vi "Test - Draw Teapot.vi"() -> ()   [LabVIEW 2022 SP3, in "Raster.lvlib"] (continued)
3"={"Position"={"x"=314.33466, "y"=375.0982, "z"=0.9916978}, "UV"={"u"=0.0, "v"=0.0}, "Colour"=12517256}, "Alpha"=0.0, "Alpha Blending Enabled"=FALSE, "Colour"=10409073}, {"Vertex 1"={"Position"={"x"=470.44748, "y"=365.30457, "z"=0.99189657}, "UV"={"u"=0.0, "v"=0.0}, "Colour"=12517256}, "Vertex 2"={"Position"={"x"=469.86905, "y"=368.43405, "z"=0.9918814}, "UV"={"u"=0.0, "v"=0.0}, "Colour"=12517256}, "Vertex 3"={"Position"={"x"=485.44525, "y"=370.00763, "z"=0.99169356}, "UV"={"u"=0.0, "v"=0.0}, "Colour"=12517256}, "Alpha"=0.0, "Alpha Blending Enabled"=FALSE, "Colour"=2964768}, {"Vertex 1"={"Position"={"x"=469.71655, "y"=372.48022, "z"=0.9918774}, "UV"={"u"=0.0, "v"=0.0}, "Colour"=12517256}, "Vertex 2"={"Position"={"x"=470.04498, "y"=373.40598, "z"=0.991886}, "UV"={"u"=0.0, "v"=0.0}, "Colour"=12517256}, "Vertex 3"={"Position"={"x"=485.66537, "y"=375.0982, "z"=0.9916978}, "UV"={"u"=0.0, "v"=0.0}, "Colour"=12517256}, "Alpha"=0.0, "Alpha Blending Enabled"=FALSE, "Colour"=10540914}, {"Vertex 1"={"Position"={"x"=329.95502, "y"=373.40598, "z"=0.991886}, "UV"={"u"=0.0, "v"=0.0}, "Colour"=12517256}, "Vertex 2"={"Position"={"x"=330.28342, "y"=372.48022, "z"=0.9918774}, "UV"={"u"=0.0, "v"=0.0}, "Colour"=12517256}, "Vertex 3"={"Position"={"x"=314.74542, "y"=374.1431, "z"=0.9916899}, "UV"={"u"=0.0, "v"=0.0}, "Colour"=12517256}, "Alpha"=0.0, "Alpha Blending Enabled"=FALSE, "Colour"=10540914}, {"Vertex 1"={"Position"={"x"=330.35867, "y"=370.8254, "z"=0.9918754}, "UV"={"u"=0.0, "v"=0.0}, "Colour"=12517256}, "Vertex 2"={"Position"={"x"=330.13095, "y"=368.43405, "z"=0.9918814}, "UV"={"u"=0.0, "v"=0.0}, "Colour"=12517256}, "Vertex 3"={"Position"={"x"=314.55475, "y"=370.00763, "z"=0.99169356}, "UV"={"u"=0.0, "v"=0.0}, "Colour"=12517256}, "Alpha"=0.0, "Alpha Blending Enabled"=FALSE, "Colour"=4875061}, {"Vertex 1"={"Position"={"x"=469.86905, "y"=368.43405, "z"=0.9918814}, "UV"={"u"=0.0, "v"=0.0}, "Colour"=12517256}, "Vertex 2"={"Position"={"x"=469.6413, "y"=370.8254, "z"=0.9918754}, "UV"={"u"=0.0, "v"=0.0}, "Colour"=12517256}, "Vertex 3"={"Position"={"x"=485.16046, "y"=372.44852, "z"=0.9916881}, "UV"={"u"=0.0, "v"=0.0}, "Colour"=12517256}, "Alpha"=0.0, "Alpha Blending Enabled"=FALSE, "Colour"=4875061}, {"Vertex 1"={"Position"={"x"=469.6413, "y"=370.8254, "z"=0.9918754}, "UV"={"u"=0.0, "v"=0.0}, "Colour"=12517256}, "Vertex 2"={"Position"={"x"=469.71655, "y"=372.48022, "z"=0.9918774}, "UV"={"u"=0.0, "v"=0.0}, "Colour"=12517256}, "Vertex 3"={"Position"={"x"=485.25458, "y"=374.1431, "z"=0.9916899}, "UV"={"u"=0.0, "v"=0.0}, "Colour"=12517256}, "Alpha"=0.0, "Alpha Blending Enabled"=FALSE, "Colour"=7510354}, {"Vertex 1"={"Position"={"x"=330.28342, "y"=372.48022, "z"=0.9918774}, "UV"={"u"=0.0, "v"=0.0}, "Colour"=12517256}, "Vertex 2"={"Position"={"x"=330.35867, "y"=370.8254, "z"=0.9918754}, "UV"={"u"=0.0, "v"=0.0}, "Colour"=12517256}, "Vertex 3"={"Position"={"x"=314.83954, "y"=372.44852, "z"=0.9916881}, "UV"={"u"=0.0, "v"=0.0}, "Colour"=12517256}, "Alpha"=0.0, "Alpha Blending Enabled"=FALSE, "Colour"=7510354}, {"Vertex 1"={"Position"={"x"=314.33466, "y"=375.0982, "z"=0.9916978}, "UV"={"u"=0.0, "v"=0.0}, "Colour"=12517256}, "Vertex 2"={"Position"={"x"=313.6705, "y"=375.32452, "z"=0.9917106}, "UV"={"u"=0.0, "v"=0.0}, "Colour"=12517256}, "Vertex 3"={"Position"={"x"=329.42438, "y"=373.61435, "z"=0.99189997}, "UV"={"u"=0.0, "v"=0.0}, "Colour"=12517256}, "Alpha"=0.0, "Alpha Blending Enabled"=FALSE, "Colour"=10409073}, {"Vertex 1"={"Position"={"x"=485.44525, "y"=370.00763, "z"=0.99169356}, "UV"={"u"=0.0, "v"=0.0}, "Colour"=12517256}, "Vertex 2"={"Position"={"x"=486.1691, "y"=366.81888, "z"=0.9917075}, "UV"={"u"=0.0, "v"=0.0}, "Colour"=12517256}, "Vertex 3"={"Position"={"x"=470.44748, "y"=365.30457, "z"=0.99189657}, "UV"={"u"=0.0, "v"=0.0}, "Colour"=12517256}, "Alpha"=0.0, "Alpha Blending Enabled"=FALSE, "Colour"=2964768}, {"Vertex 1"={"Position"={"x"=486.3295, "y"=375.32452, "z"=0.9917106}, "UV"={"u"=0.0, "v"=0.0}, "Colour"=12517256}, "Vertex 2"={"Position"={"x"=485.66537, "y"=375.0982, "z"=0.9916978}, "UV"={"u"=0.0, "v"=0.0}, "Colour"=12517256}, "Vertex 3"={"Position"={"x"=470.04498, "y"=373.40598, "z"=0.991886}, "UV"={"u"=0.0, "v"=0.0}, "Colour"=12517256}, "Alpha"=0.0, "Alpha Blending Enabled"=FALSE, "Colour"=10409073}, {"Vertex 1"={"Position"={"x"=313.8309, "y"=366.81888, "z"=0.9917075}, "UV"={"u"=0.0, "v"=0.0}, "Colour"=12517256}, "Vertex 2"={"Position"={"x"=314.55475, "y"=370.00763, "z"=0.99169356}, "UV"={"u"=0.0, "v"=0.0}, "Colour"=12517256}, "Vertex 3"={"Position"={"x"=330.13095, "y"=368.43405, "z"=0.9918814}, "UV"={"u"=0.0, "v"=0.0}, "Colour"=12517256}, "Alpha"=0.0, "Alpha Blending Enabled"=FALSE, "Colour"=2964768}, {"Vertex 1"={"Position"={"x"=314.74542, "y"=374.1431, "z"=0.9916899}, "UV"={"u"=0.0, "v"=0.0}, "Colour"=12517256}, "Vertex 2"={"Position"={"x"=314.33466, "y"=375.0982, "z"=0.9916978}, "UV"={"u"=0.0, "v"=0.0}, "Colour"=12517256}, "Vertex 3"={"Position"={"x"=329.95502, "y"=373.40598, "z"=0.991886}, "UV"={"u"=0.0, "v"=0.0}, "Colour"=12517256}, "Alpha"=0.0, "Alpha Blending Enabled"=FALSE, "Colour"=10540658}, {"Vertex 1"={"Position"={"x"=485.66537, "y"=375.0982, "z"=0.9916978}, "UV"={"u"=0.0, "v"=0.0}, "Colour"=12517256}, "Vertex 2"={"Position"={"x"=485.25458, "y"=374.1431, "z"=0.9916899}, "UV"={"u"=0.0, "v"=0.0}, "Colour"=12517256}, "Vertex 3"={"Position"={"x"=469.71655, "y"=372.48022, "z"=0.9918774}, "UV"={"u"=0.0, "v"=0.0}, "Colour"=12517256}, "Alpha"=0.0, "Alpha Blending Enabled"=FALSE, "Colour"=10540658}, {"Vertex 1"={"Position"={"x"=485.16046, "y"=372.44852, "z"=0.9916881}, "UV"={"u"=0.0, "v"=0.0}, "Colour"=12517256}, "Vertex 2"={"Position"={"x"=485.44525, "y"=370.00763, "z"=0.99169356}, "UV"={"u"=0.0, "v"=0.0}, "Colour"=12517256}, "Vertex 3"={"Position"={"x"=469.86905, "y"=368.43405, "z"=0.9918814}, "UV"={"u"=0.0, "v"=0.0}, "Colour"=12517256}, "Alpha"=0.0, "Alpha Blending Enabled"=FALSE, "Colour"=4875061}, {"Vertex 1"={"Position"={"x"=314.55475, "y"=370.00763, "z"=0.99169356}, "UV"={"u"=0.0, "v"=0.0}, "Colour"=12517256}, "Vertex 2"={"Position"={"x"=314.83954, "y"=372.44852, "z"=0.9916881}, "UV"={"u"=0.0, "v"=0.0}, "Colour"=12517256}, "Vertex 3"={"Position"={"x"=330.35867, "y"=370.8254, "z"=0.9918754}, "UV"={"u"=0.0, "v"=0.0}, "Colour"=12517256}, "Alpha"=0.0, "Alpha Blending Enabled"=FALSE, "Colour"=4875061}, {"Vertex 1"={"Position"={"x"=314.83954, "y"=372.44852, "z"=0.9916881}, "UV"={"u"=0.0, "v"=0.0}, "Colour"=12517256}, "Vertex 2"={"Position"={"x"=314.74542, "y"=374.1431, "z"=0.9916899}, "UV"={"u"=0.0, "v"=0.0}, "Colour"=12517256}, "Vertex 3"={"Position"={"x"=330.28342, "y"=372.48022, "z"=0.9918774}, "UV"={"u"=0.0, "v"=0.0}, "Colour"=12517256}, "Alpha"=0.0, "Alpha Blending Enabled"=FALSE, "Colour"=7510354}, {"Vertex 1"={"Position"={"x"=485.25458, "y"=374.1431, "z"=0.9916899}, "UV"={"u"=0.0, "v"=0.0}, "Colour"=12517256}, "Vertex 2"={"Position"={"x"=485.16046, "y"=372.44852, "z"=0.9916881}, "UV"={"u"=0.0, "v"=0.0}, "Colour"=12517256}, "Vertex 3"={"Position"={"x"=469.6413, "y"=370.8254, "z"=0.9918754}, "UV"={"u"=0.0, "v"=0.0}, "Colour"=12517256}, "Alpha"=0.0, "Alpha Blending Enabled"=FALSE, "Colour"=7510354}, {"Vertex 1"={"Position"={"x"=485.66537, "y"=375.0982, "z"=0.9916978}, "UV"={"u"=0.0, "v"=0.0}, "Colour"=12517256}, "Vertex 2"={"Position"={"x"=486.3295, "y"=375.32452, "z"=0.9917106}, "UV"={"u"=0.0, "v"=0.0}, "Colour"=12517256}, "Vertex 3"={"Position"={"x"=501.1485, "y"=377.42767, "z"=0.9914777}, "UV"={"u"=0.0, "v"=0.0}, "Colour"=12517256}, "Alpha"=0.0, "Alpha Blending Enabled"=FALSE, "Colour"=10145646}, {"Vertex 1"={"Position"={"x"=314.55475, "y"=370.00763, "z"=0.99169356}, "UV"={"u"=0.0, "v"=0.0}, "Colour"=12517256}, "Vertex 2"={"Position"={"x"=313.8309, "y"=366.81888, "z"=0.9917075}, "UV"={"u"=0.0, "v"=0.0}, "Colour"=12517256}, "Vertex 3"={"Position"={"x"=299.04465, "y"=368.681, "z"=0.991475}, "UV"={"u"=0.0, "v"=0.0}, "Colour"=12517256}, "Alpha"=0.0, "Alpha Blending Enabled"=FALSE, "Colour"=2107927}, {"Vertex 1"={"Position"={"x"=313.6705, "y"=375.32452, "z"=0.9917106}, "UV"={"u"=0.0, "v"=0.0}, "Colour"=12517256}, "Vertex 2"={"Position"={"x"=314.33466, "y"=375.0982, "z"=0.9916978}, "UV"={"u"=0.0, "v"=0.0}, "Colour"=12517256}, "Vertex 3"={"Position"={"x"=299.65118, "y"=377.17847, "z"=0.99146646}, "UV"={"u"=0.0, "v"=0.0}, "Colour"=12517256}, "Alpha"=0.0, "Alpha Blending Enabled"=FALSE, "Colour"=10145646}, {"Vertex 1"={"Position"={"x"=486.1691, "y"=366.81888, "z"=0.9917075}, "UV"={"u"=0.0, "v"=0.0}, "Colour"=12517256}, "Vertex 2"={"Position"={"x"=485.44525, "y"=370.00763, "z"=0.99169356}, "UV"={"u"=0.0, "v"=0.0}, "Colour"=12517256}, "Vertex 3"={"Position"={"x"=500.08383, "y"=371.94174, "z"=0.9914627}, "UV"={"u"=0.0, "v"=0.0}, "Colour"=12517256}, "Alpha"=0.0, "Alpha Blending Enabled"=FALSE, "Colour"=2107927}, {"Vertex 1"={"Position"={"x"=485.25458, "y"=374.1431, "z"=0.9916899}, "UV"={"u"=0.0, "v"=0.0}, "Colour"=12517256}, "Vertex 2"={"Position"={"x"=485.66537, "y"=375.0982, "z"=0.9916978}, "UV"={"u"=0.0, "v"=0.0}, "Colour"=12517256}, "Vertex 3"={"Position"={"x"=500.34882, "y"=377.17847, "z"=0.99146646}, "UV"={"u"=0.0, "v"=0.0}, "Colour"=12517256}, "Alpha"=0.0, "Alpha Blending Enabled"=FALSE, "Colour"=9750122}, {"Vertex 1"={"Position"={"x"=314.33466, "y"=375.0982, "z"=0.9916978}, "UV"={"u"=0.0, "v"=0.0}, "Colour"=12517256}, "Vertex 2"={"Position"={"x"=314.74542, "y"=374.1431, "z"=0.9916899}, "UV"={"u"=0.0, "v"=0.0}, "Colour"=12517256}, "Vertex 3"={"Position"={"x"=300.14566, "y"=376.18677, "z"=0.9914595}, "UV"={"u"=0.0, "v"=0.0}, "Colour"=12517256}, "Alpha"=0.0, "Alpha Blending Enabled"=FALSE, "Colour"=9750122}, {"Vertex 1"={"Position"={"x"=314.83954, "y"=372.44852, "z"=0.9916881}, "UV"={"u"=0.0, "v"=0.0}, "Colour"=12517256}, "Vertex 2"={"Position"={"x"=314.55475, "y"=370.00763, "z"=0.99169356}, "UV"={"u"=0.0, "v"=0.0}, "Colour"=12517256}, "Vertex 3"={"Position"={"x"=299.91617, "y"=371.94174, "z"=0.9914627}, "UV"={"u"=0.0, "v"=0.0}, "Colour"=12517256}, "Alpha"=0.0, "Alpha Blending Enabled"=FALSE, "Colour"=3886890}, {"Vertex 1"={"Position"={"x"=485.44525, "y"=370.00763, "z"=0.99169356}, "UV"={"u"=0.0, "v"=0.0}, "Colour"=12517256}, "Vertex 2"={"Position"={"x"=485.16046, "y"=372.44852, "z"=0.9916881}, "UV"={"u"=0.0, "v"=0.0}, "Colour"=12517256}, "Vertex 3"={"Position"={"x"=499.7411, "y"=374.4432, "z"=0.9914579}, "UV"={"u"=0.0, "v"=0.0}, "Colour"=12517256}, "Alpha"=0.0, "Alpha Blending Enabled"=FALSE, "Colour"=3886890}, {"Vertex 1"={"Position"={"x"=485.16046, "y"=372.44852, "z"=0.9916881}, "UV"={"u"=0.0, "v"=0.0}, "Colour"=12517256}, "Vertex 2"={"Position"={"x"=485.25458, "y"=374.1431, "z"=0.9916899}, "UV"={"u"=0.0, "v"=0.0}, "Colour"=12517256}, "Vertex 3"={"Position"={"x"=499.85434, "y"=376.18677, "z"=0.9914595}, "UV"={"u"=0.0, "v"=0.0}, "Colour"=12517256}, "Alpha"=0.0, "Alpha Blending Enabled"=FALSE, "Colour"=6522183}, {"Vertex 1"={"Position"={"x"=314.74542, "y"=374.1431, "z"=0.9916899}, "UV"={"u"=0.0, "v"=0.0}, "Colour"=12517256}, "Vertex 2"={"Position"={"x"=314.83954, "y"=372.44852, "z"=0.9916881}, "UV"={"u"=0.0, "v"=0.0}, "Colour"=12517256}, "Vertex 3"={"Position"={"x"=300.2589, "y"=374.4432, "z"=0.9914579}, "UV"={"u"=0.0, "v"=0.0}, "Colour"=12517256}, "Alpha"=0.0, "Alpha Blending Enabled"=FALSE, "Colour"=6522183}, {"Vertex 1"={"Position"={"x"=299.65118, "y"=377.17847, "z"=0.99146646}, "UV"={"u"=0.0, "v"=0.0}, "Colour"=12517256}, "Vertex 2"={"Position"={"x"=298.8515, "y"=377.42767, "z"=0.9914777}, "UV"={"u"=0.0, "v"=0.0}, "Colour"=12517256}, "Vertex 3"={"Position"={"x"=313.6705, "y"=375.32452, "z"=0.9917106}, "UV"={"u"=0.0, "v"=0.0}, "Colour"=12517256}, "Alpha"=0.0, "Alpha Blending Enabled"=FALSE, "Colour"=10145646}, {"Vertex 1"={"Position"={"x"=500.08383, "y"=371.94174, "z"=0.9914627}, "UV"={"u"=0.0, "v"=0.0}, "Colour"=12517256}, "Vertex 2"={"Position"={"x"=500.95535, "y"=368.681, "z"=0.991475}, "UV"={"u"=0.0, "v"=0.0}, "Colour"=12517256}, "Vertex 3"={"Position"={"x"=486.1691, "y"=366.81888, "z"=0.9917075}, "UV"={"u"=0.0, "v"=0.0}, "Colour"=12517256}, "Alpha"=0.0, "Alpha Blending Enabled"=FALSE, "Colour"=2107927}, {"Vertex 1"={"Position"={"x"=501.1485, "y"=377.42767, "z"=0.9914777}, "UV"={"u"=0.0, "v"=0.0}, "Colour"=12517256}, "Vertex 2"={"Position"={"x"=500.34882, "y"=377.17847, "z"=0.99146646}, "UV"={"u"=0.0, "v"=0.0}, "Colour"=12517256}, "Vertex 3"={"Position"={"x"=485.66537, "y"=375.0982, "z"=0.9916978}, "UV"={"u"=0.0, "v"=0.0}, "Colour"=12517256}, "Alpha"=0.0, "Alpha Blending Enabled"=FALSE, "Colour"=10145646}, {"Vertex 1"={"Position"={"x"=299.04465, "y"=368.681, "z"=0.991475}, "UV"={"u"=0.0, "v"=0.0}, "Colour"=12517256}, "Vertex 2"={"Position"={"x"=299.91617, "y"=371.94174, "z"=0.9914627}, "UV"={"u"=0.0, "v"=0.0}, "Colour"=12517256}, "Vertex 3"={"Position"={"x"=314.55475, "y"=370.00763, "z"=0.99169356}, "UV"={"u"=0.0, "v"=0.0}, "Colour"=12517256}, "Alpha"=0.0, "Alpha Blending Enabled"=FALSE, "Colour"=2107927}, {"Vertex 1"={"Position"={"x"=300.14566, "y"=376.18677, "z"=0.9914595}, "UV"={"u"=0.0, "v"=0.0}, "Colour"=12517256}, "Vertex 2"={"Position"={"x"=299.65118, "y"=377.17847, "z"=0.99146646}, "UV"={"u"=0.0, "v"=0.0}, "Colour"=12517256}, "Vertex 3"={"Position"={"x"=314.33466, "y"=375.0982, "z"=0.9916978}, "UV"={"u"=0.0, "v"=0.0}, "Colour"=12517256}, "Alpha"=0.0, "Alpha Blending Enabled"=FALSE, "Colour"=9750122}, {"Vertex 1"={"Position"={"x"=500.34882, "y"=377.17847, "z"=0.99146646}, "UV"={"u"=0.0, "v"=0.0}, "Colour"=12517256}, "Vertex 2"={"Position"={"x"=499.85434, "y"=376.18677, "z"=0.9914595}, "UV"={"u"=0.0, "v"=0.0}, "Colour"=12517256}, "Vertex 3"={"Position"={"x"=485.25458, "y"=374.1431, "z"=0.9916899}, "UV"={"u"=0.0, "v"=0.0}, "Colour"=12517256}, "Alpha"=0.0, "Alpha Blending Enabled"=FALSE, "Colour"=9750122}, {"Vertex 1"={"Position"={"x"=499.7411, "y"=374.4432, "z"=0.9914579}, "UV"={"u"=0.0, "v"=0.0}, "Colour"=12517256}, "Vertex 2"={"Position"={"x"=500.08383, "y"=371.94174, "z"=0.9914627}, "UV"={"u"=0.0, "v"=0.0}, "Colour"=12517256}, "Vertex 3"={"Position"={"x"=485.44525, "y"=370.00763, "z"=0.99169356}, "UV"={"u"=0.0, "v"=0.0}, "Colour"=12517256}, "Alpha"=0.0, "Alpha Blending Enabled"=FALSE, "Colour"=3886890}, {"Vertex 1"={"Position"={"x"=299.91617, "y"=371.94174, "z"=0.9914627}, "UV"={"u"=0.0, "v"=0.0}, "Colour"=12517256}, "Vertex 2"={"Position"={"x"=300.2589, "y"=374.4432, "z"=0.9914579}, "UV"={"u"=0.0, "v"=0.0}, "Colour"=12517256}, "Vertex 3"={"Position"={"x"=314.83954, "y"=372.44852, "z"=0.9916881}, "UV"={"u"=0.0, "v"=0.0}, "Colour"=12517256}, "Alpha"=0.0, "Alpha Blending Enabled"=FALSE, "Colour"=3886890}, {"Vertex 1"={"Position"={"x"=300.2589, "y"=374.4432, "z"=0.9914579}, "UV"={"u"=0.0, "v"=0.0}, "Colour"=12517256}, "Vertex 2"={"Position"={"x"=300.14566, "y"=376.18677, "z"=0.9914595}, "UV"={"u"=0.0, "v"=0.0}, "Colour"=12517256}, "Vertex 3"={"Position"={"x"=314.74542, "y"=374.1431, "z"=0.9916899}, "UV"={"u"=0.0, "v"=0.0}, "Colour"=12517256}, "Alpha"=0.0, "Alpha Blending Enabled"=FALSE, "Colour"=6522183}, {"Vertex 1"={"Position"={"x"=499.85434, "y"=376.18677, "z"=0.9914595}, "UV"={"u"=0.0, "v"=0.0}, "Colour"=12517256}, "Vertex 2"={"Position"={"x"=499.7411, "y"=374.4432, "z"=0.9914579}, "UV"={"u"=0.0, "v"=0.0}, "Colour"=12517256}, "Vertex 3"={"Position"={"x"=485.16046, "y"=372.44852, "z"=0.9916881}, "UV"={"u"=0.0, "v"=0.0}, "Colour"=12517256}, "Alpha"=0.0, "Alpha Blending Enabled"=FALSE, "Colour"=6522183}, {"Vertex 1"={"Position"={"x"=500.34882, "y"=377.17847, "z"=0.99146646}, "UV"={"u"=0.0, "v"=0.0}, "Colour"=12517256}, "Vertex 2"={"Position"={"x"=501.1485, "y"=377.42767, "z"=0.9914777}, "UV"={"u"=0.0, "v"=0.0}, "Colour"=12517256}, "Vertex 3"={"Position"={"x"=514.8347, "y"=379.946, "z"=0.9911989}, "UV"={"u"=0.0, "v"=0.0}, "Colour"=12517256}, "Alpha"=0.0, "Alpha Blending Enabled"=FALSE, "Colour"=9816171}, {"Vertex 1"={"Position"={"x"=299.91617, "y"=371.94174, "z"=0.9914627}, "UV"={"u"=0.0, "v"=0.0}, "Colour"=12517256}, "Vertex 2"={"Position"={"x"=299.04465, "y"=368.681, "z"=0.991475}, "UV"={"u"=0.0, "v"=0.0}, "Colour"=12517256}, "Vertex 3"={"Position"={"x"=285.39166, "y"=370.91043, "z"=0.9911967}, "UV"={"u"=0.0, "v"=0.0}, "Colour"=12517256}, "Alpha"=0.0, "Alpha Blending Enabled"=FALSE, "Colour"=1053963}, {"Vertex 1"={"Position"={"x"=298.8515, "y"=377.42767, "z"=0.9914777}, "UV"={"u"=0.0, "v"=0.0}, "Colour"=12517256}, "Vertex 2"={"Position"={"x"=299.65118, "y"=377.17847, "z"=0.99146646}, "UV"={"u"=0.0, "v"=0.0}, "Colour"=12517256}, "Vertex 3"={"Position"={"x"=286.10245, "y"=379.66818, "z"=0.9911896}, "UV"={"u"=0.0, "v"=0.0}, "Colour"=12517256}, "Alpha"=0.0, "Alpha Blending Enabled"=FALSE, "Colour"=9816171}, {"Vertex 1"={"Position"={"x"=500.95535, "y"=368.681, "z"=0.991475}, "UV"={"u"=0.0, "v"=0.0}, "Colour"=12517256}, "Vertex 2"={"Position"={"x"=500.08383, "y"=371.94174, "z"=0.9914627}, "UV"={"u"=0.0, "v"=0.0}, "Colour"=12517256}, "Vertex 3"={"Position"={"x"=513.58716, "y"=374.2562, "z"=0.99118644}, "UV"={"u"=0.0, "v"=0.0}, "Colour"=12517256}, "Alpha"=0.0, "Alpha Blending Enabled"=FALSE, "Colour"=1053963}, {"Vertex 1"={"Position"={"x"=499.85434, "y"=376.18677, "z"=0.9914595}, "UV"={"u"=0.0, "v"=0.0}, "Colour"=12517256}, "Vertex 2"={"Position"={"x"=500.34882, "y"=377.17847, "z"=0.99146646}, "UV"={"u"=0.0, "v"=0.0}, "Colour"=12517256}, "Vertex 3"={"Position"={"x"=513.8976, "y"=379.66818, "z"=0.9911896}, "UV"={"u"=0.0, "v"=0.0}, "Colour"=12517256}, "Alpha"=0.0, "Alpha Blending Enabled"=FALSE, "Colour"=8827744}, {"Vertex 1"={"Position"={"x"=299.65118, "y"=377.17847, "z"=0.99146646}, "UV"={"u"=0.0, "v"=0.0}, "Colour"=12517256}, "Vertex 2"={"Position"={"x"=300.14566, "y"=376.18677, "z"=0.9914595}, "UV"={"u"=0.0, "v"=0.0}, "Colour"=12517256}, "Vertex 3"={"Position"={"x"=286.68176, "y"=378.632, "z"=0.99118376}, "UV"={"u"=0.0, "v"=0.0}, "Colour"=12517256}, "Alpha"=0.0, "Alpha Blending Enabled"=FALSE, "Colour"=8827744}, {"Vertex 1"={"Position"={"x"=300.2589, "y"=374.4432, "z"=0.9914579}, "UV"={"u"=0.0, "v"=0.0}, "Colour"=12517256}, "Vertex 2"={"Position"={"x"=299.91617, "y"=371.94174, "z"=0.9914627}, "UV"={"u"=0.0, "v"=0.0}, "Colour"=12517256}, "Vertex 3"={"Position"={"x"=286.41284, "y"=374.2562, "z"=0.99118644}, "UV"={"u"=0.0, "v"=0.0}, "Colour"=12517256}, "Alpha"=0.0, "Alpha Blending Enabled"=FALSE, "Colour"=2832670}, {"Vertex 1"={"Position"={"x"=500.08383, "y"=371.94174, "z"=0.9914627}, "UV"={"u"=0.0, "v"=0.0}, "Colour"=12517256}, "Vertex 2"={"Position"={"x"=499.7411, "y"=374.4432, "z"=0.9914579}, "UV"={"u"=0.0, "v"=0.0}, "Colour"=12517256}, "Vertex 3"={"Position"={"x"=513.18567, "y"=376.82974, "z"=0.99118245}, "UV"={"u"=0.0, "v"=0.0}, "Colour"=12517256}, "Alpha"=0.0, "Alpha Blending Enabled"=FALSE, "Colour"=2832670}, {"Vertex 1"={"Position"={"x"=499.7411, "y"=374.4432, "z"=0.9914579}, "UV"={"u"=0.0, "v"=0.0}, "Colour"=12517256}, "Vertex 2"={"Position"={"x"=499.85434, "y"=376.18677, "z"=0.9914595}, "UV"={"u"=0.0, "v"=0.0}, "Colour"=12517256}, "Vertex 3"={"Position"={"x"=513.31824, "y"=378.632, "z"=0.99118376}, "UV"={"u"=0.0, "v"=0.0}, "Colour"=12517256}, "Alpha"=0.0, "Alpha Blending Enabled"=FALSE, "Colour"=5467963}, {"Vertex 1"={"Position"={"x"=300.14566, "y"=376.18677, "z"=0.9914595}, "UV"={"u"=0.0, "v"=0.0}, "Colour"=12517256}, "Vertex 2"={"Position"={"x"=300.2589, "y"=374.4432, "z"=0.9914579}, "UV"={"u"=0.0, "v"=0.0}, "Colour"=12517256}, "Vertex 3"={"Position"={"x"=286.81436, "y"=376.82974, "z"=0.99118245}, "UV"={"u"=0.0, "v"=0.0}, "Colour"=12517256}, "Alpha"=0.0, "Alpha Blending Enabled"=FALSE, "Colour"=5467963}, {"Vertex 1"={"Position"={"x"=286.10245, "y"=379.66818, "z"=0.9911896}, "UV"={"u"=0.0, "v"=0.0}, "Colour"=12517256}, "Vertex 2"={"Position"={"x"=285.16525, "y"=379.946, "z"=0.9911989}, "UV"={"u"=0.0, "v"=0.0}, "Colour"=12517256}, "Vertex 3"={"Position"={"x"=298.8515, "y"=377.42767, "z"=0.9914777}, "UV"={"u"=0.0, "v"=0.0}, "Colour"=12517256}, "Alpha"=0.0, "Alpha Blending Enabled"=FALSE, "Colour"=9816171}, {"Vertex 1"={"Position"={"x"=513.58716, "y"=374.2562, "z"=0.99118644}, "UV"={"u"=0.0, "v"=0.0}, "Colour"=12517256}, "Vertex 2"={"Position"={"x"=514.60834, "y"=370.91043, "z"=0.9911967}, "UV"={"u"=0.0, "v"=0.0}, "Colour"=12517256}, "Vertex 3"={"Position"={"x"=500.95535, "y"=368.681, "z"=0.991475}, "UV"={"u"=0.0, "v"=0.0}, "Colour"=12517256}, "Alpha"=0.0, "Alpha Blending Enabled"=FALSE, "Colour"=1053963}, {"Vertex 1"={"Position"={"x"=514.8347, "y"=379.946, "z"=0.9911989}, "UV"={"u"=0.0, "v"=0.0}, "Colour"=12517256}, "Vertex 2"={"Position"={"x"=513.8976, "y"=379.66818, "z"=0.9911896}, "UV"={"u"=0.0, "v"=0.0}, "Colour"=12517256}, "Vertex 3"={"Position"={"x"=500.34882, "y"=377.17847, "z"=0.99146646}, "UV"={"u"=0.0, "v"=0.0}, "Colour"=12517256}, "Alpha"=0.0, "Alpha Blending Enabled"=FALSE, "Colour"=9816171}, {"Vertex 1"={"Position"={"x"=285.39166, "y"=370.91043, "z"=0.9911967}, "UV"={"u"=0.0, "v"=0.0}, "Colour"=12517256}, "Vertex 2"={"Position"={"x"=286.41284, "y"=374.2562, "z"=0.99118644}, "UV"={"u"=0.0, "v"=0.0}, "Colour"=12517256}, "Vertex 3"={"Position"={"x"=299.91617, "y"=371.94174, "z"=0.9914627}, "UV"={"u"=0.0, "v"=0.0}, "Colour"=12517256}, "Alpha"=0.0, "Alpha Blending Enabled"=FALSE, "Colour"=1053963}, {"Vertex 1"={"Position"={"x"=286.68176, "y"=378.632, "z"=0.99118376}, "UV"={"u"=0.0, "v"=0.0}, "Colour"=12517256}, "Vertex 2"={"Position"={"x"=286.10245, "y"=379.66818, "z"=0.9911896}, "UV"={"u"=0.0, "v"=0.0}, "Colour"=12517256}, "Vertex 3"={"Position"={"x"=299.65118, "y"=377.17847, "z"=0.99146646}, "UV"={"u"=0.0, "v"=0.0}, "Colour"=12517256}, "Alpha"=0.0, "Alpha Blending Enabled"=FALSE, "Colour"=8827744}, {"Vertex 1"={"Position"={"x"=513.8976, "y"=379.66818, "z"=0.9911896}, "UV"={"u"=0.0, "v"=0.0}, "Colour"=12517256}, "Vertex 2"={"Position"={"x"=513.31824, "y"=378.632, "z"=0.99118376}, "UV"={"u"=0.0, "v"=0.0}, "Colour"=12517256}, "Vertex 3"={"Position"={"x"=499.85434, "y"=376.18677, "z"=0.9914595}, "UV"={"u"=0.0, "v"=0.0}, "Colour"=12517256}, "Alpha"=0.0, "Alpha Blending Enabled"=FALSE, "Colour"=8827744}, {"Vertex 1"={"Position"={"x"=513.18567, "y"=376.82974, "z"=0.99118245}, "UV"={"u"=0.0, "v"=0.0}, "Colour"=12517256}, "Vertex 2"={"Position"={"x"=513.58716, "y"=374.2562, "z"=0.99118644}, "UV"={"u"=0.0, "v"=0.0}, "Colour"=12517256}, "Vertex 3"={"Position"={"x"=500.08383, "y"=371.94174, "z"=0.9914627}, "UV"={"u"=0.0, "v"=0.0}, "Colour"=12517256}, "Alpha"=0.0, "Alpha Blending Enabled"=FALSE, "Colour"=2832670}, {"Vertex 1"={"Position"={"x"=286.41284, "y"=374.2562, "z"=0.99118644}, "UV"={"u"=0.0, "v"=0.0}, "Colour"=12517256}, "Vertex 2"={"Position"={"x"=286.81436, "y"=376.82974, "z"=0.99118245}, "UV"={"u"=0.0, "v"=0.0}, "Colour"=12517256}, "Vertex 3"={"Position"={"x"=300.2589, "y"=374.4432, "z"=0.9914579}, "UV"={"u"=0.0, "v"=0.0}, "Colour"=12517256}, "Alpha"=0.0, "Alpha Blending Enabled"=FALSE, "Colour"=2832670}, {"Vertex 1"={"Position"={"x"=286.81436, "y"=376.82974, "z"=0.99118245}, "UV"={"u"=0.0, "v"=0.0}, "Colour"=12517256}, "Vertex 2"={"Position"={"x"=286.68176, "y"=378.632, "z"=0.99118376}, "UV"={"u"=0.0, "v"=0.0}, "Colour"=12517256}, "Vertex 3"={"Position"={"x"=300.14566, "y"=376.18677, "z"=0.9914595}, "UV"={"u"=0.0, "v"=0.0}, "Colour"=12517256}, "Alpha"=0.0, "Alpha Blending Enabled"=FALSE, "Colour"=5467963}, {"Vertex 1"={"Position"={"x"=513.31824, "y"=378.632, "z"=0.99118376}, "UV"={"u"=0.0, "v"=0.0}, "Colour"=12517256}, "Vertex 2"={"Position"={"x"=513.18567, "y"=376.82974, "z"=0.99118245}, "UV"={"u"=0.0, "v"=0.0}, "Colour"=12517256}, "Vertex 3"={"Position"={"x"=499.7411, "y"=374.4432, "z"=0.9914579}, "UV"={"u"=0.0, "v"=0.0}, "Colour"=12517256}, "Alpha"=0.0, "Alpha Blending Enabled"=FALSE, "Colour"=5467963}, {"Vertex 1"={"Position"={"x"=513.8976, "y"=379.66818, "z"=0.9911896}, "UV"={"u"=0.0, "v"=0.0}, "Colour"=12517256}, "Vertex 2"={"Position"={"x"=514.8347, "y"=379.946, "z"=0.9911989}, "UV"={"u"=0.0, "v"=0.0}, "Colour"=12517256}, "Vertex 3"={"Position"={"x"=527.11084, "y"=382.90955, "z"=0.99087083}, "UV"={"u"=0.0, "v"=0.0}, "Colour"=12517256}, "Alpha"=0.0, "Alpha Blending Enabled"=FALSE, "Colour"=9486695}, {"Vertex 1"={"Position"={"x"=285.16525, "y"=379.946, "z"=0.9911989}, "UV"={"u"=0.0, "v"=0.0}, "Colour"=12517256}, "Vertex 2"={"Position"={"x"=286.10245, "y"=379.66818, "z"=0.9911896}, "UV"={"u"=0.0, "v"=0.0}, "Colour"=12517256}, "Vertex 3"={"Position"={"x"=273.96463, "y"=382.5964, "z"=0.9908639}, "UV"={"u"=0.0, "v"=0.0}, "Colour"=12517256}, "Alpha"=0.0, "Alpha Blending Enabled"=FALSE, "Colour"=9486695}, {"Vertex 1"={"Position"={"x"=286.41284, "y"=374.2562, "z"=0.99118644}, "UV"={"u"=0.0, "v"=0.0}, "Colour"=12517256}, "Vertex 2"={"Position"={"x"=285.39166, "y"=370.91043, "z"=0.9911967}, "UV"={"u"=0.0, "v"=0.0}, "Colour"=12517256}, "Vertex 3"={"Position"={"x"=273.14902, "y"=373.53363, "z"=0.99086916}, "UV"={"u"=0.0, "v"=0.0}, "Colour"=12517256}, "Alpha"=0.0, "Alpha Blending Enabled"=FALSE, "Colour"=131841}, {"Vertex 1"={"Position"={"x"=514.60834, "y"=370.91043, "z"=0.9911967}, "UV"={"u"=0.0, "v"=0.0}, "Colour"=12517256}, "Vertex 2"={"Position"={"x"=513.58716, "y"=374.2562, "z"=0.99118644}, "UV"={"u"=0.0, "v"=0.0}, "Colour"=12517256}, "Vertex 3"={"Position"={"x"=525.67926, "y"=376.97778, "z"=0.99086154}, "UV"={"u"=0.0, "v"=0.0}, "Colour"=12517256}, "Alpha"=0.0, "Alpha Blending Enabled"=FALSE, "Colour"=131841}, {"Vertex 1"={"Position"={"x"=513.31824, "y"=378.632, "z"=0.99118376}, "UV"={"u"=0.0, "v"=0.0}, "Colour"=12517256}, "Vertex 2"={"Position"={"x"=513.8976, "y"=379.66818, "z"=0.9911896}, "UV"={"u"=0.0, "v"=0.0}, "Colour"=12517256}, "Vertex 3"={"Position"={"x"=526.03534, "y"=382.5964, "z"=0.9908639}, "UV"={"u"=0.0, "v"=0.0}, "Colour"=12517256}, "Alpha"=0.0, "Alpha Blending Enabled"=FALSE, "Colour"=7773780}, {"Vertex 1"={"Position"={"x"=286.10245, "y"=379.66818, "z"=0.9911896}, "UV"={"u"=0.0, "v"=0.0}, "Colour"=12517256}, "Vertex 2"={"Position"={"x"=286.68176, "y"=378.632, "z"=0.99118376}, "UV"={"u"=0.0, "v"=0.0}, "Colour"=12517256}, "Vertex 3"={"Position"={"x"=274.62903, "y"=381.50693, "z"=0.99085957}, "UV"={"u"=0.0, "v"=0.0}, "Colour"=12517256}, "Alpha"=0.0, "Alpha Blending Enabled"=FALSE, "Colour"=7773780}, {"Vertex 1"={"Position"={"x"=286.81436, "y"=376.82974, "z"=0.99118245}, "UV"={"u"=0.0, "v"=0.0}, "Colour"=12517256}, "Vertex 2"={"Position"={"x"=286.41284, "y"=374.2562, "z"=0.99118644}, "UV"={"u"=0.0, "v"=0.0}, "Colour"=12517256}, "Vertex 3"={"Position"={"x"=274.32074, "y"=376.97778, "z"=0.99086154}, "UV"={"u"=0.0, "v"=0.0}, "Colour"=12517256}, "Alpha"=0.0, "Alpha Blending Enabled"=FALSE, "Colour"=1581329}, {"Vertex 1"={"Position"={"x"=513.58716, "y"=374.2562, "z"=0.99118644}, "UV"={"u"=0.0, "v"=0.0}, "Colour"=12517256}, "Vertex 2"={"Position"={"x"=513.18567, "y"=376.82974, "z"=0.99118245}, "UV"={"u"=0.0, "v"=0.0}, "Colour"=12517256}, "Vertex 3"={"Position"={"x"=525.2189, "y"=379.6353, "z"=0.99085855}, "UV"={"u"=0.0, "v"=0.0}, "Colour"=12517256}, "Alpha"=0.0, "Alpha Blending Enabled"=FALSE, "Colour"=1581329}, {"Vertex 1"={"Position"={"x"=513.18567, "y"=376.82974, "z"=0.99118245}, "UV"={"u"=0.0, "v"=0.0}, "Colour"=12517256}, "Vertex 2"={"Position"={"x"=513.31824, "y"=378.632, "z"=0.99118376}, "UV"={"u"=0.0, "v"=0.0}, "Colour"=12517256}, "Vertex 3"={"Position"={"x"=525.371, "y"=381.50693, "z"=0.99085957}, "UV"={"u"=0.0, "v"=0.0}, "Colour"=12517256}, "Alpha"=0.0, "Alpha Blending Enabled"=FALSE, "Colour"=4216366}, {"Vertex 1"={"Position"={"x"=286.68176, "y"=378.632, "z"=0.99118376}, "UV"={"u"=0.0, "v"=0.0}, "Colour"=12517256}, "Vertex 2"={"Position"={"x"=286.81436, "y"=376.82974, "z"=0.99118245}, "UV"={"u"=0.0, "v"=0.0}, "Colour"=12517256}, "Vertex 3"={"Position"={"x"=274.78113, "y"=379.6353, "z"=0.99085855}, "UV"={"u"=0.0, "v"=0.0}, "Colour"=12517256}, "Alpha"=0.0, "Alpha Blending Enabled"=FALSE, "Colour"=4216366}, {"Vertex 1"={"Position"={"x"=273.96463, "y"=382.5964, "z"=0.9908639}, "UV"={"u"=0.0, "v"=0.0}, "Colour"=12517256}, "Vertex 2"={"Position"={"x"=272.88913, "y"=382.90955, "z"=0.99087083}, "UV"={"u"=0.0, "v"=0.0}, "Colour"=12517256}, "Vertex 3"={"Position"={"x"=285.16525, "y"=379.946, "z"=0.9911989}, "UV"={"u"=0.0, "v"=0.0}, "Colour"=12517256}, "Alpha"=0.0, "Alpha Blending Enabled"=FALSE, "Colour"=9486695}, {"Vertex 1"={"Position"={"x"=525.67926, "y"=376.97778, "z"=0.99086154}, "UV"={"u"=0.0, "v"=0.0}, "Colour"=12517256}, "Vertex 2"={"Position"={"x"=526.851, "y"=373.53363, "z"=0.99086916}, "UV"={"u"=0.0, "v"=0.0}, "Colour"=12517256}, "Vertex 3"={"Position"={"x"=514.60834, "y"=370.91043, "z"=0.9911967}, "UV"={"u"=0.0, "v"=0.0}, "Colour"=12517256}, "Alpha"=0.0, "Alpha Blending Enabled"=FALSE, "Colour"=131841}, {"Vertex 1"={"Position"={"x"=527.11084, "y"=382.90955, "z"=0.99087083}, "UV"={"u"=0.0, "v"=0.0}, "Colour"=12517256}, "Vertex 2"={"Position"={"x"=526.03534, "y"=382.5964, "z"=0.9908639}, "UV"={"u"=0.0, "v"=0.0}, "Colour"=12517256}, "Vertex 3"={"Position"={"x"=513.8976, "y"=379.66818, "z"=0.9911896}, "UV"={"u"=0.0, "v"=0.0}, "Colour"=12517256}, "Alpha"=0.0, "Alpha Blending Enabled"=FALSE, "Colour"=9486695}, {"Vertex 1"={"Position"={"x"=273.14902, "y"=373.53363, "z"=0.99086916}, "UV"={"u"=0.0, "v"=0.0}, "Colour"=12517256}, "Vertex 2"={"Position"={"x"=274.32074, "y"=376.97778, "z"=0.99086154}, "UV"={"u"=0.0, "v"=0.0}, "Colour"=12517256}, "Vertex 3"={"Position"={"x"=286.41284, "y"=374.2562, "z"=0.99118644}, "UV"={"u"=0.0, "v"=0.0}, "Colour"=12517256}, "Alpha"=0.0, "Alpha Blending Enabled"=FALSE, "Colour"=131841}, {"Vertex 1"={"Position"={"x"=274.62903, "y"=381.50693, "z"=0.99085957}, "UV"={"u"=0.0, "v"=0.0}, "Colour"=12517256}, "Vertex 2"={"Position"={"x"=273.96463, "y"=382.5964, "z"=0.9908639}, "UV"={"u"=0.0, "v"=0.0}, "Colour"=12517256}, "Vertex 3"={"Position"={"x"=286.10245, "y"=379.66818, "z"=0.9911896}, "UV"={"u"=0.0, "v"=0.0}, "Colour"=12517256}, "Alpha"=0.0, "Alpha Blending Enabled"=FALSE, "Colour"=7773780}, {"Vertex 1"={"Position"={"x"=526.03534, "y"=382.5964, "z"=0.9908639}, "UV"={"u"=0.0, "v"=0.0}, "Colour"=12517256}, "Vertex 2"={"Position"={"x"=525.371, "y"=381.50693, "z"=0.99085957}, "UV"={"u"=0.0, "v"=0.0}, "Colour"=12517256}, "Vertex 3"={"Position"={"x"=513.31824, "y"=378.632, "z"=0.99118376}, "UV"={"u"=0.0, "v"=0.0}, "Colour"=12517256}, "Alpha"=0.0, "Alpha Blending Enabled"=FALSE, "Colour"=7773780}, {"Vertex 1"={"Position"={"x"=525.2189, "y"=379.6353, "z"=0.99085855}, "UV"={"u"=0.0, "v"=0.0}, "Colour"=12517256}, "Vertex 2"={"Position"={"x"=525.67926, "y"=376.97778, "z"=0.99086154}, "UV"={"u"=0.0, "v"=0.0}, "Colour"=12517256}, "Vertex 3"={"Position"={"x"=513.58716, "y"=374.2562, "z"=0.99118644}, "UV"={"u"=0.0, "v"=0.0}, "Colour"=12517256}, "Alpha"=0.0, "Alpha Blending Enabled"=FALSE, "Colour"=1581329}, {"Vertex 1"={"Position"={"x"=274.32074, "y"=376.97778, "z"=0.99086154}, "UV"={"u"=0.0, "v"=0.0}, "Colour"=12517256}, "Vertex 2"={"Position"={"x"=274.78113, "y"=379.6353, "z"=0.99085855}, "UV"={"u"=0.0, "v"=0.0}, "Colour"=12517256}, "Vertex 3"={"Position"={"x"=286.81436, "y"=376.82974, "z"=0.99118245}, "UV"={"u"=0.0, "v"=0.0}, "Colour"=12517256}, "Alpha"=0.0, "Alpha Blending Enabled"=FALSE, "Colour"=1581329}, {"Vertex 1"={"Position"={"x"=274.78113, "y"=379.6353, "z"=0.99085855}, "UV"={"u"=0.0, "v"=0.0}, "Colour"=12517256}, "Vertex 2"={"Position"={"x"=274.62903, "y"=381.50693, "z"=0.99085957}, "UV"={"u"=0.0, "v"=0.0}, "Colour"=12517256}, "Vertex 3"={"Position"={"x"=286.68176, "y"=378.632, "z"=0.99118376}, "UV"={"u"=0.0, "v"=0.0}, "Colour"=12517256}, "Alpha"=0.0, "Alpha Blending Enabled"=FALSE, "Colour"=4216366}, {"Vertex 1"={"Position"={"x"=525.371, "y"=381.50693, "z"=0.99085957}, "UV"={"u"=0.0, "v"=0.0}, "Colour"=12517256}, "Vertex 2"={"Position"={"x"=525.2189, "y"=379.6353, "z"=0.99085855}, "UV"={"u"=0.0, "v"=0.0}, "Colour"=12517256}, "Vertex 3"={"Position"={"x"=513.18567, "y"=376.82974, "z"=0.99118245}, "UV"={"u"=0.0, "v"=0.0}, "Colour"=12517256}, "Alpha"=0.0, "Alpha Blending Enabled"=FALSE, "Colour"=4216366}, {"Vertex 1"={"Position"={"x"=526.03534, "y"=382.5964, "z"=0.9908639}, "UV"={"u"=0.0, "v"=0.0}, "Colour"=12517256}, "Vertex 2"={"Position"={"x"=527.11084, "y"=382.90955, "z"=0.99087083}, "UV"={"u"=0.0, "v"=0.0}, "Colour"=12517256}, "Vertex 3"={"Position"={"x"=537.603, "y"=386.3562, "z"=0.99048924}, "UV"={"u"=0.0, "v"=0.0}, "Colour"=12517256}, "Alpha"=0.0, "Alpha Blending Enabled"=FALSE, "Colour"=9091427}, {"Vertex 1"={"Position"={"x"=272.88913, "y"=382.90955, "z"=0.99087083}, "UV"={"u"=0.0, "v"=0.0}, "Colour"=12517256}, "Vertex 2"={"Position"={"x"=273.96463, "y"=382.5964, "z"=0.9908639}, "UV"={"u"=0.0, "v"=0.0}, "Colour"=12517256}, "Vertex 3"={"Position"={"x"=263.60925, "y"=385.99985, "z"=0.99048537}, "UV"={"u"=0.0, "v"=0.0}, "Colour"=12517256}, "Alpha"=0.0, "Alpha Blending Enabled"=FALSE, "Colour"=9091427}, {"Vertex 1"={"Position"={"x"=274.32074, "y"=376.97778, "z"=0.99086154}, "UV"={"u"=0.0, "v"=0.0}, "Colour"=12517256}, "Vertex 2"={"Position"={"x"=273.14902, "y"=373.53363, "z"=0.99086916}, "UV"={"u"=0.0, "v"=0.0}, "Colour"=12517256}, "Vertex 3"={"Position"={"x"=262.69003, "y"=376.584, "z"=0.9904883}, "UV"={"u"=0.0, "v"=0.0}, "Colour"=12517256}, "Alpha"=0.0, "Alpha Blending Enabled"=FALSE, "Colour"=131841}, {"Vertex 1"={"Position"={"x"=526.851, "y"=373.53363, "z"=0.99086916}, "UV"={"u"=0.0, "v"=0.0}, "Colour"=12517256}, "Vertex 2"={"Position"={"x"=525.67926, "y"=376.97778, "z"=0.99086154}, "UV"={"u"=0.0, "v"=0.0}, "Colour"=12517256}, "Vertex 3"={"Position"={"x"=535.98956, "y"=380.14035, "z"=0.99048406}, "UV"={"u"=0.0, "v"=0.0}, "Colour"=12517256}, "Alpha"=0.0, "Alpha Blending Enabled"=FALSE, "Colour"=131841}, {"Vertex 1"={"Position"={"x"=525.371, "y"=381.50693, "z"=0.99085957}, "UV"={"u"=0.0, "v"=0.0}, "Colour"=12517256}, "Vertex 2"={"Position"={"x"=526.03534, "y"=382.5964, "z"=0.9908639}, "UV"={"u"=0.0, "v"=0.0}, "Colour"=12517256}, "Vertex 3"={"Position"={"x"=536.39075, "y"=385.99985, "z"=0.99048537}, "UV"={"u"=0.0, "v"=0.0}, "Colour"=12517256}, "Alpha"=0.0, "Alpha Blending Enabled"=FALSE, "Colour"=6654024}, {"Vertex 1"={"Position"={"x"=273.96463, "y"=382.5964, "z"=0.9908639}, 
